vi "Get Max Heat Capacity.vi"(8 "error in (no error)":errorcluster, 11 "VISA resource name":refnum<visa-resource-name>) -> (0 "error out":errorcluster, 1 "HeatMax (out)":i8, 3 "VISA resource name out":refnum<visa-resource-name>)   [LabVIEW 2015, in "JULABO DeviceDriver.lvlib"]
doc: "This Vi returns the maximum allowed heating capacity in percent"
uses:
  JULABO DeviceDriver.lvlib
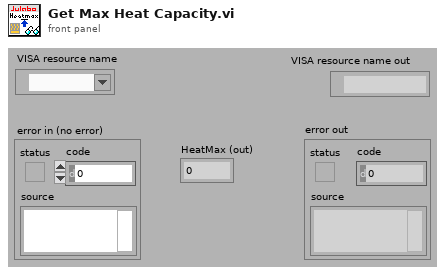
[diagram p1: front panel]
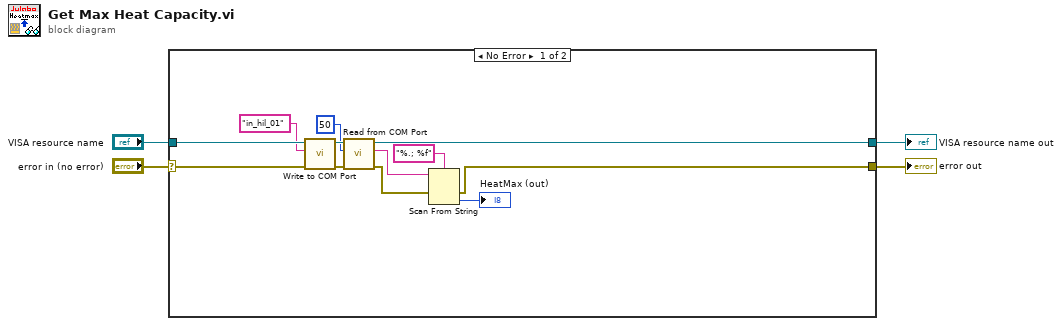
[diagram p0: block diagram]
diagram:
  n1 = case shown="No Error" "error in (no error)" {
    selector: "error in (no error)" -> [w15 w17]
    tunnel: "VISA resource name" -> [w16 w18]
    tunnel: [w14 w17] -> w2
    tunnel: [w13 w18] -> w1
    frame No Error {
      n2 = call "Write to COM Port.vi"("error in"=w15, "Command (input)"="in_hil_01", "VISA resource name in"=w16) -> ("error out"=w12:errorcluster, "VISA resource name out"=w11:refnum<visa-resource-name>)  [unwired: 7 in]
      n3 = call "Read from COM Port.vi"("error in"=w12, "Byte to Read (-1:All)"=u32 50 ("Anzahl der Byte"), "VISA resource name in"=w11) -> ("error out"=w9:errorcluster, "String (output)"=w8:string, "VISA resource name out"=w13:refnum<visa-resource-name>)  [unwired: 5 in, 1 out]
      n4 = Scan From String(format string="%.; %f" ("Format-String"), input string=w8, error in=w9) -> (error out=w14:errorcluster, output 1=→"HeatMax (out)":i8)  [unwired: 2 in, 2 out]
    }
    frame Error {
    }
  }
  "error out" <- w2
  "VISA resource name out" <- w1
